vi "Leer_FicheroConfigEstacion_XML.vi"(8 "error in (no error)":errorcluster, 11 "XML File Path":path=path "C:/Trabajo_Robot/TFG_ROBOT/CONTROL_ROBOT/LABVIEW_ROBOT_MASTER") -> (0 "error out":errorcluster, 3 "Coordenadas_estacion":T1)   [LabVIEW 2019, in "SHARED VI'S.lvlib"]
uses:
  LVPROJ_CONFIG_ESTACION/Type_defs/Coordenadas_estacion.ctl
  <vilib>/Utility/xml.llb/Read From XML File(string).vi
  SHARED VI'S.lvlib
panel:
  out "XML Elements":string
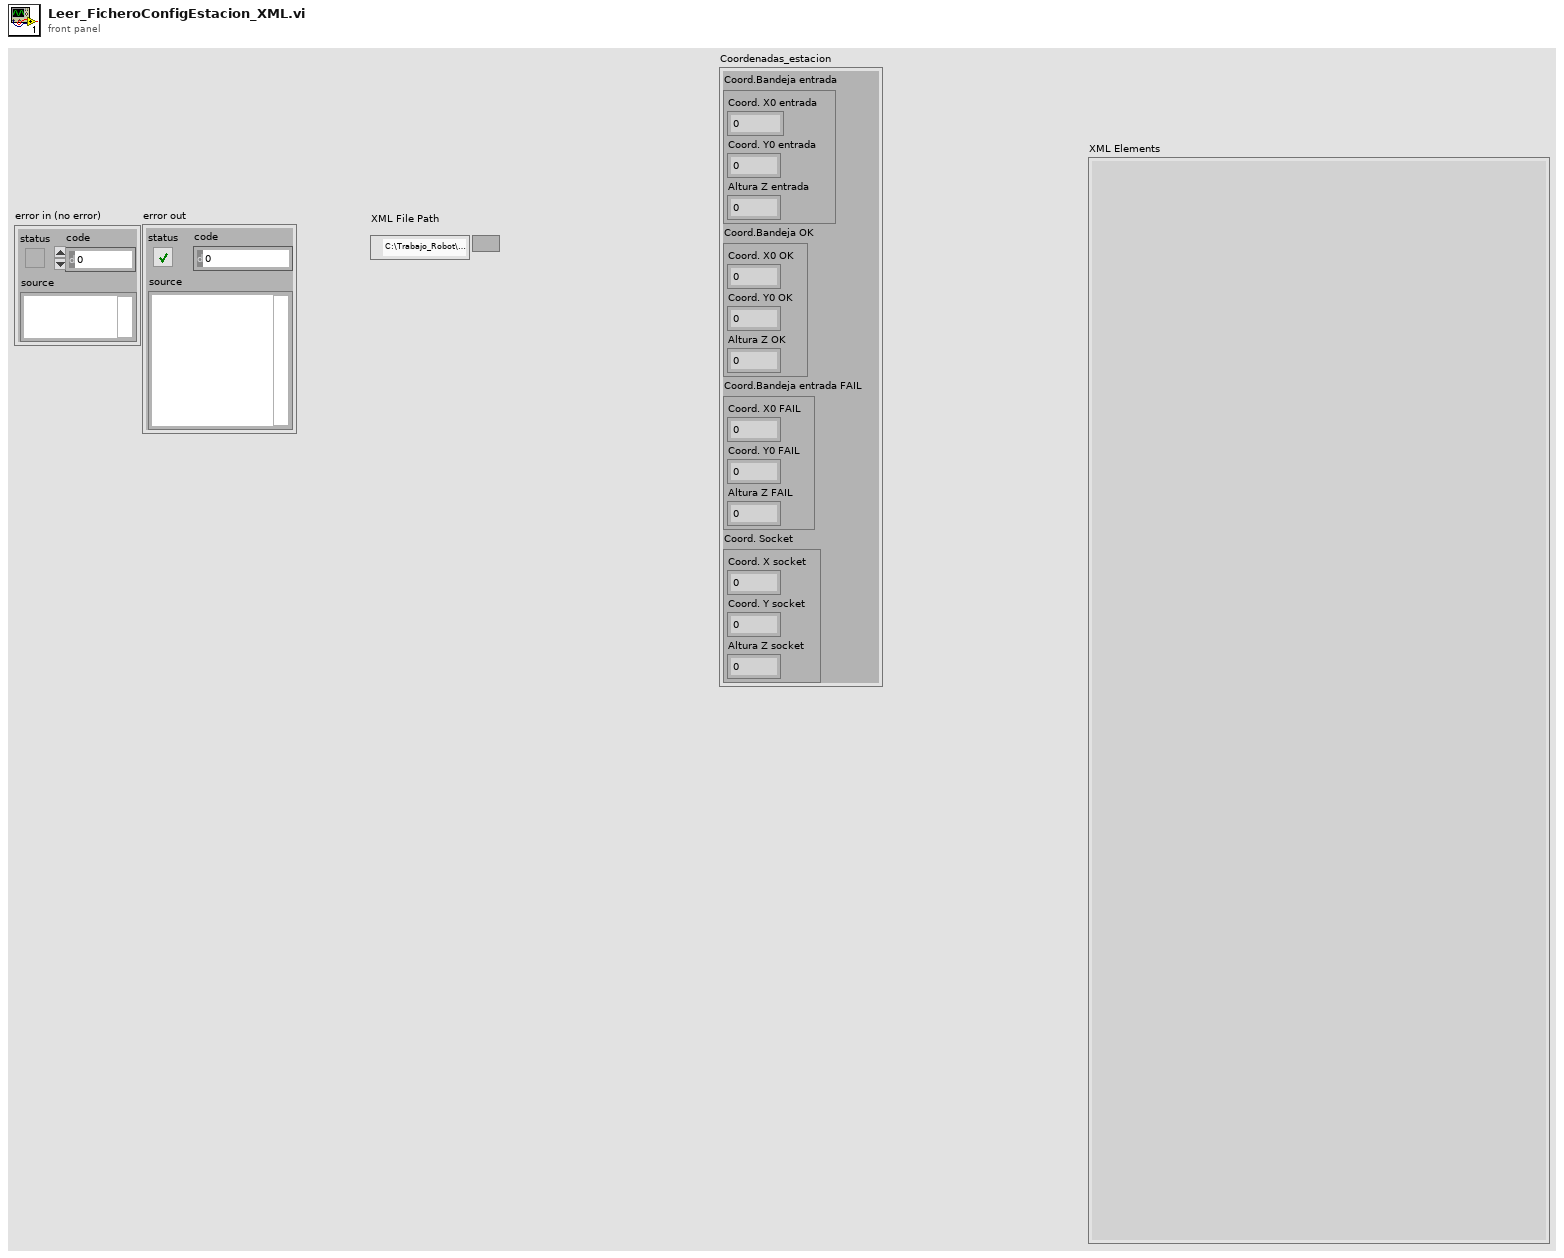
[diagram p1: front panel]
types:
  T1 = typedef "Coordenadas_estacion.ctl" = cluster{"Coord.Bandeja entrada":cluster{"Coord. X0 entrada":u32, "Coord. Y0 entrada ":u32, "Altura Z entrada":u32}, "Coord.Bandeja OK":cluster{"Coord. X0 OK":u32, "Coord. Y0 OK":u32, "Altura Z OK":u32}, "Coord.Bandeja entrada FAIL":cluster{"Coord. X0 FAIL":u32, "Coord. Y0 FAIL":u32, "Altura Z FAIL":u32}, "Coord. Socket":cluster{"Coord. X socket":u32, "Coord. Y socket":u32, "Altura Z socket":u32}}
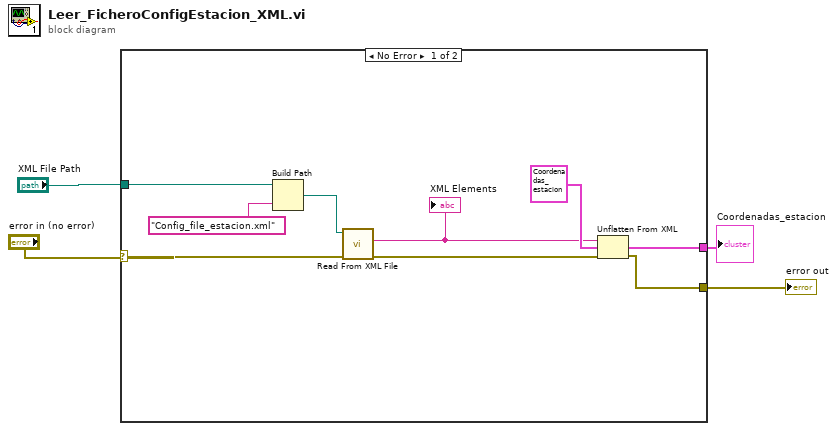
[diagram p0: block diagram]
diagram:
  n1 = case shown="No Error" "error in (no error)" {
    selector: "error in (no error)" -> [w10 _]
    tunnel: [w9 _] -> w3
    tunnel: [w8 _] -> w2
    tunnel: "XML File Path" -> [w7 _]
    frame No Error {
      n2 = Build Path(base path=w7, name or relative path="Config_file_estacion.xml") -> (appended path=w5:path)
      n3 = call-poly <vilib>:"Read From XML File.vi"("error in (no error)"=w10, "XML File Path"=w5) -> ("error out"=w11:errorcluster, "XML Elements"=w12:string)  [unwired: 7 in, 1 out]
      "XML Elements" <- w12
      n4 = Unflatten From XML(xml string=w12, type=T1 {"Coord.Bandeja entrada"={"Coord. X0 entrada"=0, "Coord. Y0 entrada "=0, "Altura Z entrada"=0}, "Coord.Bandeja OK"={"Coord. X0 OK"=0, "Coord. Y0 OK"=0, "Altura Z OK"=0}, "Coord.Bandeja entrada FAIL"={"Coord. X0 FAIL"=0, "Coord. Y0 FAIL"=0, "Altura Z FAIL"=0}, "Coord. Socket"={"Coord. X socket"=0, "Coord. Y socket"=0, "Altura Z socket"=0}} ("Coordenadas_estacion"), error in (no error)=w11) -> (value=w8:T1, error out=w9:errorcluster)
    }
    frame Error {
    }
  }
  "error out" <- w3
  "Coordenadas_estacion" <- w2
